vi "n set input pointer.vi"(8 "error in (no error)":errorcluster, 10 "pointer":i32, 11 "n":u16) -> (0 "error out":errorcluster)   [LabVIEW 2015, in "SCANalone4x64.lvlib"]
doc: "__declspec(dllimport) void __stdcall n_set_input_pointer(unsigned short n, long pointer);"
uses:
  <userlib>/SCANalone4x64/SCANalone4x64.lvlib
  <userlib>/SCANalone4x64/SCANalone4x64.dll
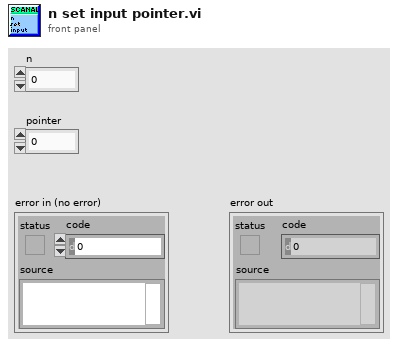
[diagram p1: front panel]
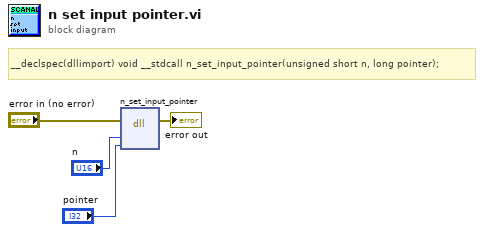
[diagram p0: block diagram]
diagram:
  # "__declspec(dllimport) void __stdcall n_set_input_pointer(unsigned short n, long pointer);"
  n1 = dll-call lib="C:/Program Files/National Instruments/LabVIEW 2015/user.lib/SCANalone4x64/SCANalone4x64.*" fn="n_set_input_pointer"(error in="error in (no error)", "n"="n", "pointer"="pointer") -> (error out=→"error out":errorcluster)  [unwired: 5 in, 1 out]
